vi "SW_Gen_Get_Bounding_rectangles.vi"(10 "Radius of displayed outer segments, pix":dbl, 11 "Draw Area Size":cluster{"Width":dbl, "Height":dbl}) -> (3 "Bounding rectangle for outer segments":T1)   [LabVIEW 2016]
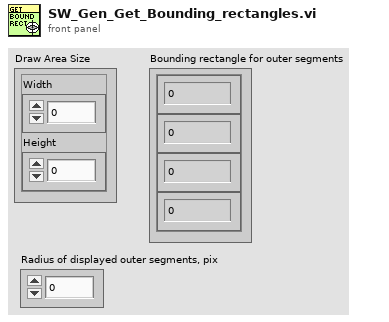
[diagram p1: front panel]
types:
  T1 = cluster{"Numeric Control":dbl, "Numeric Control":dbl, "Numeric Control":dbl, "Numeric Control":dbl}
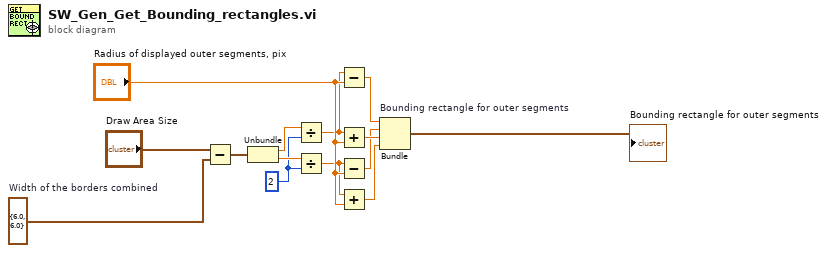
[diagram p0: block diagram]
diagram:
  w9 = cluster{"Width":dbl, "Height":dbl} {"Width"=6.0, "Height"=6.0}  # Width of the borders combined
  w2 = u32 2 ("y")
  n1 = Subtract(x="Draw Area Size", y=w9) -> (x-y=w10:cluster{"Width":dbl, "Height":dbl})
  n2 = Unbundle(w10) -> ("Width"=w12:dbl, "Height"=w13:dbl)
  n3 = Divide(x=w12, y=w2) -> (x/y=w3:dbl)
  n4 = Divide(x=w13, y=w2) -> (x/y=w4:dbl)
  n5 = Subtract(x=w3, y="Radius of displayed outer segments, pix") -> (x-y=w5:dbl)
  n6 = Add(x=w3, y="Radius of displayed outer segments, pix") -> (x+y=w7:dbl)
  n7 = Subtract(x=w4, y="Radius of displayed outer segments, pix") -> (x-y=w6:dbl)
  n8 = Add(x=w4, y="Radius of displayed outer segments, pix") -> (x+y=w8:dbl)
  n9 = Bundle "Bounding rectangle for outer segments"(w5, w6, w7, w8) -> (→"Bounding rectangle for outer segments":cluster{dbl, dbl, dbl, dbl})  [unwired: 1 in]
